vi "Shutdown DUT.vi"(7 "0x01 (F)":bool, 8 "error in (no error)":errorcluster, 9 "Device On?":bool, 10 "Blast?":bool, 11 "Data In":T1={"Message"="", "Homed?"=FALSE, "NextState"=enum."Timeout", "G.Load"=0.0, "G.Position"=0.0, "Load#"=0, "[G.Loads]"=[], "[TotalLoads]"=[], "[Errors]"=[], "ZeroWait"=0, "Results"=[], "DwellWait"=FALSE, "Test Result"=FALSE, "[CondyleLoads]"=[], "[Max]"=[], "[Min]"=[], "Valid String?"=FALSE, "ScanTime"=timestamp(0 s since 1904-01-01), "ScannedString"="", "LabelDevID"=0, "MfgDate"=timestamp(0 s since 1904-01-01), "[EEPROM Cmds]"=[], "[CalData]"=[], "[A/Ds]"=[], "[A/Dmax]"=[], "[A/Dmin]"=[], "BattMax"=0.0, "BattMin"=0.0, "DwellTime"=2000, "PendingDeviceType"="", "Zero G.load"=0.0, "GAINC Value"="", "Programming Step"=enum."Load EEPROM", "Front Panel Program?"=FALSE, "Final Program?"=FALSE, "PCB Score"=100, "AssyScore"=100, "Pass/Fail #"="", "Result String"="", "Programming Mode"=enum."Initial Program", "Angle Test Step"=enum."Initialize", "Accel Values"=[], "Shutdown Counter"=0, "V1"=0, "V2"=0, "V3"=0, "V4"=0, "EEPROM Data"=[], "Counter"=0, "Page#"=0, "Timer"=timestamp(0 s since 1904-01-01), "Use Mark10?"=FALSE, "Eng-Result#"=0, "DUT Serial #"=0, "Scroll Message?"=FALSE, "Clear Message"=FALSE, "Batt Test Step "=enum."Initialize", "RXTX Window Found?"=FALSE, "Shutdown First Call?"=FALSE, "A2 Delay (msec)"=500, "Support Script"={"Script #"="", "Script Revision"="", "[OEMs]"=[], "[[DeviceTypes]]"=[], "[[DeviceTypesVals]]"=[], "[[List of Errors]]"=[], "Default GAINC"="", "[[ASICtrims]]"=[], "ID For Echo"="", "Condyle A CalFactor"=100, "Condyle B CalFactor"=100, "[OEMs Prefix]"=[], "Packet ID 18"="", "[[Force Table Load Test]]"=[], "[[Force Table AccurTest]]"=[]}, "Serial Table"={"Serial File Path"=path "", "[[Serial Lookup Table]]"=[], "Serial Device Info"=[], "Valid Serial?"=FALSE}, "Target Information"={"Target Brand"="", "Target DeviceType"="", "Target Serial#"=100, "Target Lot#"=0, "Target DevID"=0, "Target Channel"=5}, "Operator"="", "COM Port"="", "Config Path"=path "", "Tx Array"=[], "DUT Parameters"={"Channel"=0, "DeviceID"=0, "Script Rev"=0, "Month"=0, "Day"=0, "Year"=0, "Lot#"=0, "V1"=0, "V2"=0, "V3"=0, "V4"=0, "MFG"=0, "Cal FactorA 10"=0, "Cal FactorB 10  "=0, "Cal FactorA 16"=0, "Cal FactorB 16"=0, "ASICtrim"=[], "TmpChan"=0, "GAINC"="", "Brand"="", "Device"="", "Serial #"=0, "Batt310"=0, "Batt 280"=0}, "FTS Main?"=FALSE, "Loading"={"[Forces]"=[], "[Dwell]"=[], "Loading Step"=enum."Initialize Test"}, "Software Version"="", "Correction Factor"="", "Second Load Test"=FALSE, "Acc Loads"=[], "Mark10 Config"={"H2S%"=[80.0, 85.0, 90.0, 95.0, 100.0], "H2S Speed"=[12.0, 8.0, 6.0, 4.0, 2.0], "H to S"=2.0, "Home Speed"=1.0, "LoadWin"=0.0, "Load Speed"=0.0, "PID"={"Kp"=0.04, "Kd"=0.005001, "Ki"=2.9999999999999923e-05}}, "Channels"={"Transceiver Ch"=5, "Operating Ch"=5, "Start Ch"=0}, "Channel EEPROM"=[], "Load Notes"=[], "Engr Log?"=FALSE, "Time"=[], "Program Retry"=FALSE, "Operator Channel"="", "Target Channel "="", "New Data Program"=FALSE, "NFHU Pass?"=FALSE, "Cycle Number"=0, "Cal Cycle#"=0, "[Avg G.Loads] "=[], "[Avg A/Ds] "=[], "Cal Retry?"=FALSE, "[Total A/Ds]  "=[], "Cycle Num LA"=0, "LA Cycle# "=0, "Shim Num"=0, "Shim#  "=0, "Angle Test?"=FALSE} {"Mark10 Config"."PID"."Ki" min=0.0 max=200.0 format="%.6f"; "Mark10 Config"."PID"."Kd" min=0.0 max=200.0 format="%.6f"; "Mark10 Config"."PID"."Kp" min=0.0 max=200.0 format="%.6f"; "DUT Parameters"."ASICtrim" format="%02x"}) -> (0 "error out":errorcluster, 3 "State-machine Local Variables out":T1={"Message"="", "Homed?"=FALSE, "NextState"=enum."Timeout", "G.Load"=0.0, "G.Position"=0.0, "Load#"=0, "[G.Loads]"=[], "[TotalLoads]"=[], "[Errors]"=[], "ZeroWait"=0, "Results"=[], "DwellWait"=FALSE, "Test Result"=FALSE, "[CondyleLoads]"=[], "[Max]"=[], "[Min]"=[], "Valid String?"=FALSE, "ScanTime"=timestamp(0 s since 1904-01-01), "ScannedString"="", "LabelDevID"=0, "MfgDate"=timestamp(0 s since 1904-01-01), "[EEPROM Cmds]"=[], "[CalData]"=[], "[A/Ds]"=[], "[A/Dmax]"=[], "[A/Dmin]"=[], "BattMax"=0.0, "BattMin"=0.0, "DwellTime"=2000, "PendingDeviceType"="", "Zero G.load"=0.0, "GAINC Value"="", "Programming Step"=enum."Load EEPROM", "Front Panel Program?"=FALSE, "Final Program?"=FALSE, "PCB Score"=100, "AssyScore"=100, "Pass/Fail #"="", "Result String"="", "Programming Mode"=enum."Initial Program", "Angle Test Step"=enum."Initialize", "Accel Values"=[], "Shutdown Counter"=0, "V1"=0, "V2"=0, "V3"=0, "V4"=0, "EEPROM Data"=[], "Counter"=0, "Page#"=0, "Timer"=timestamp(0 s since 1904-01-01), "Use Mark10?"=FALSE, "Eng-Result#"=0, "DUT Serial #"=0, "Scroll Message?"=FALSE, "Clear Message"=FALSE, "Batt Test Step "=enum."Initialize", "RXTX Window Found?"=FALSE, "Shutdown First Call?"=FALSE, "A2 Delay (msec)"=500, "Support Script"={"Script #"="", "Script Revision"="", "[OEMs]"=[], "[[DeviceTypes]]"=[], "[[DeviceTypesVals]]"=[], "[[List of Errors]]"=[], "Default GAINC"="", "[[ASICtrims]]"=[], "ID For Echo"="", "Condyle A CalFactor"=100, "Condyle B CalFactor"=100, "[OEMs Prefix]"=[], "Packet ID 18"="", "[[Force Table Load Test]]"=[], "[[Force Table AccurTest]]"=[]}, "Serial Table"={"Serial File Path"=path "", "[[Serial Lookup Table]]"=[], "Serial Device Info"=[], "Valid Serial?"=FALSE}, "Target Information"={"Target Brand"="", "Target DeviceType"="", "Target Serial#"=100, "Target Lot#"=0, "Target DevID"=0, "Target Channel"=5}, "Operator"="", "COM Port"="", "Config Path"=path "", "Tx Array"=[], "DUT Parameters"={"Channel"=0, "DeviceID"=0, "Script Rev"=0, "Month"=0, "Day"=0, "Year"=0, "Lot#"=0, "V1"=0, "V2"=0, "V3"=0, "V4"=0, "MFG"=0, "Cal FactorA 10"=0, "Cal FactorB 10  "=0, "Cal FactorA 16"=0, "Cal FactorB 16"=0, "ASICtrim"=[], "TmpChan"=0, "GAINC"="", "Brand"="", "Device"="", "Serial #"=0, "Batt310"=0, "Batt 280"=0}, "FTS Main?"=FALSE, "Loading"={"[Forces]"=[], "[Dwell]"=[], "Loading Step"=enum."Initialize Test"}, "Software Version"="", "Correction Factor"="", "Second Load Test"=FALSE, "Acc Loads"=[], "Mark10 Config"={"H2S%"=[80.0, 85.0, 90.0, 95.0, 100.0], "H2S Speed"=[12.0, 8.0, 6.0, 4.0, 2.0], "H to S"=2.0, "Home Speed"=1.0, "LoadWin"=0.0, "Load Speed"=0.0, "PID"={"Kp"=0.04, "Kd"=0.005001, "Ki"=2.9999999999999923e-05}}, "Channels"={"Transceiver Ch"=5, "Operating Ch"=5, "Start Ch"=0}, "Channel EEPROM"=[], "Load Notes"=[], "Engr Log?"=FALSE, "Time"=[], "Program Retry"=FALSE, "Operator Channel"="", "Target Channel "="", "New Data Program"=FALSE, "NFHU Pass?"=FALSE, "Cycle Number"=0, "Cal Cycle#"=0, "[Avg G.Loads] "=[], "[Avg A/Ds] "=[], "Cal Retry?"=FALSE, "[Total A/Ds]  "=[], "Cycle Num LA"=0, "LA Cycle# "=0, "Shim Num"=0, "Shim#  "=0, "Angle Test?"=FALSE} {"Mark10 Config"."PID"."Ki" min=0.0 max=200.0 format="%.6f"; "Mark10 Config"."PID"."Kd" min=0.0 max=200.0 format="%.6f"; "Mark10 Config"."PID"."Kp" min=0.0 max=200.0 format="%.6f"; "DUT Parameters"."ASICtrim" format="%02x"})   [LabVIEW 2015]
uses:
  Controls/LocalVars.ctl
  Controls/Gen2 FT states.ctl
  Controls/Iniial Device Programming.ctl
  ProgramStageControl.ctl
  Controls/Batt Cap Steps.ctl
  Controls/Support Script.ctl
  Controls/Serial Table.ctl
  Controls/Device Information.ctl
  Controls/InfoPacket.ctl
  Controls/Loading.ctl
  Controls/Load Step.ctl
  Controls/Mark10 Config.ctl
  Controls/PID parameters.ctl
  Controls/Channels.ctl
  RxTx/XceiverCmds.ctl
  Controls/Gen2 FT Globals.vi
panel:
  out "Numeric":i32
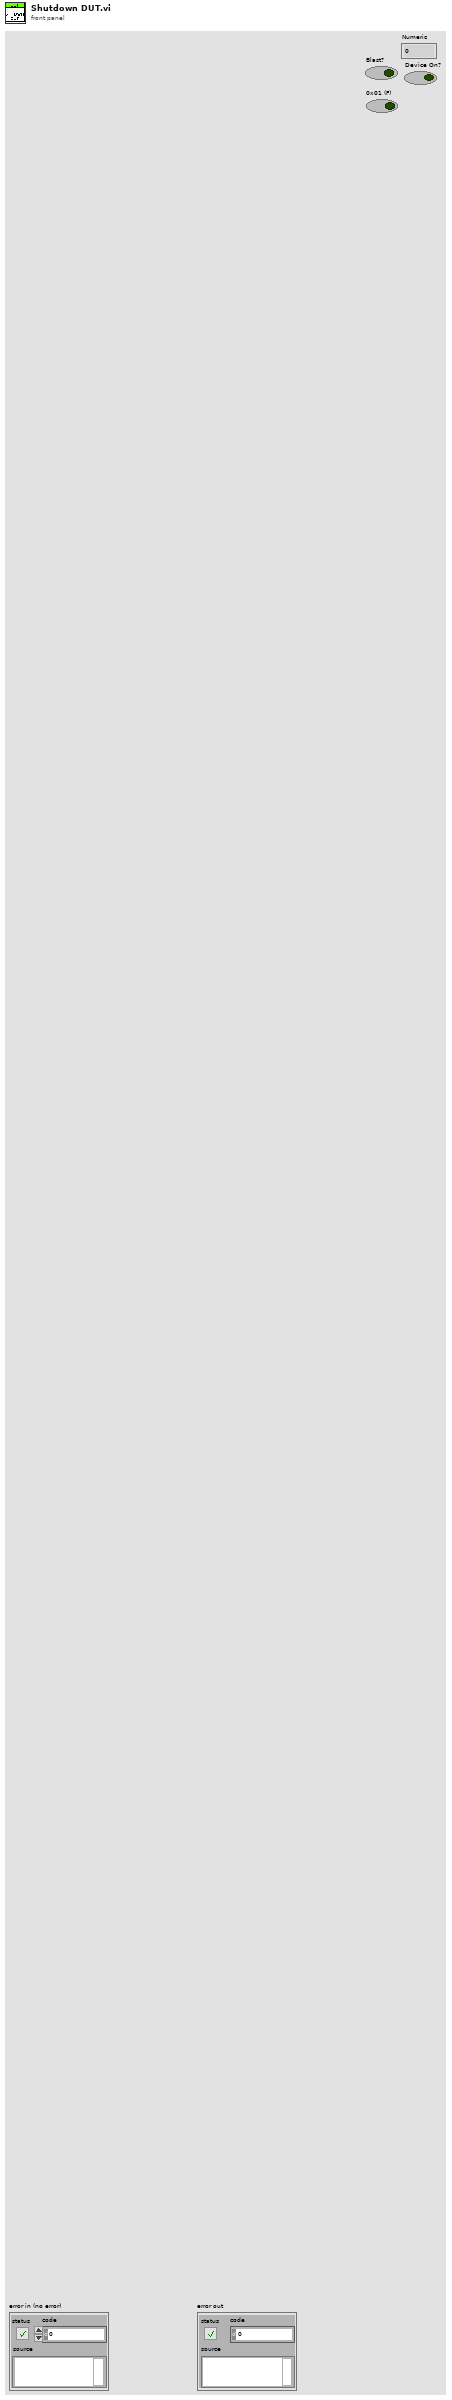
[diagram p1: front panel]
types:
  T1 = typedef "LocalVars.ctl" = cluster{"Message":string, "Homed?":bool, "NextState":T2, "G.Load":dbl, "G.Position":dbl, "Load#":i32, "[G.Loads]":dbl[], "[TotalLoads]":dbl[], "[Errors]":dbl[][], "ZeroWait":u32, "Results":dbl[], "DwellWait":bool, "Test Result":bool, "[CondyleLoads]":dbl[][], "[Max]":dbl[], "[Min]":dbl[], "Valid String?":bool, "ScanTime":timestamp, "ScannedString":string, "LabelDevID":u32, "MfgDate":timestamp, "[EEPROM Cmds]":u8[][], "[CalData]":u8[][], "[A/Ds]":dbl[][], "[A/Dmax]":dbl[], "[A/Dmin]":dbl[], "BattMax":dbl, "BattMin":dbl, "DwellTime":i32, "PendingDeviceType":string, "Zero G.load":dbl, "GAINC Value":string, "Programming Step":T3, "Front Panel Program?":bool, "Final Program?":bool, "PCB Score":i32, "AssyScore":i32, "Pass/Fail #":string, "Result String":string, "Programming Mode":T4, "Angle Test Step":enum16{"Initialize", "Get X", "Get Y", "Get Z", "Next Test"}, "Accel Values":dbl[][], "Shutdown Counter":u32, "V1":i32, "V2":i32, "V3":i32, "V4":i32, "EEPROM Data":i32[][], "Counter":i32, "Page#":i32, "Timer":timestamp, "Use Mark10?":bool, "Eng-Result#":u32, "DUT Serial #":i32, "Scroll Message?":bool, "Clear Message":bool, "Batt Test Step ":T5, "RXTX Window Found?":bool, "Shutdown First Call?":bool, "A2 Delay (msec)":i16, "Support Script":T6, "Serial Table":T7, "Target Information":T8, "Operator":string, "COM Port":string, "Config Path":path, "Tx Array":u8[], "DUT Parameters":T9, "FTS Main?":bool, "Loading":T10, "Software Version":string, "Correction Factor":string, "Second Load Test":bool, "Acc Loads":dbl[][], "Mark10 Config":T12, "Channels":T14, "Channel EEPROM":i32[][], "Load Notes":string[], "Engr Log?":bool, "Time":timestamp[], "Program Retry":bool, "Operator Channel":string, "Target Channel ":string, "New Data Program":bool, "NFHU Pass?":bool, "Cycle Number":i32, "Cal Cycle#":i32, "[Avg G.Loads] ":dbl[], "[Avg A/Ds] ":dbl[][], "Cal Retry?":bool, "[Total A/Ds]  ":dbl[][], "Cycle Num LA":i32, "LA Cycle# ":i32, "Shim Num":i32, "Shim#  ":i32, "Angle Test?":bool}
  T2 = typedef "Gen2 FT states.ctl" = enum16{"---------SETUP-------", "Initialization", "Read Support Data", "Initialize Mark-10", "Initialize Transceiver", "------UTILITIES------", "Change DUT Channel", "Find RxTx Window", "Reset Device", "Scan Channels", "Read Serial Lookup", "Shutdown Device", "ESTOP", "--------USER---------", "Timeout", "-----PROGRAM-----", "Program Device", "------MARK10--------", "Go Home", "MoveUp", "MoveDown", "Goto Load", "Goto Position", "Stop Motor", "---------TESTS--------", "Start Test", "Angle Test", "Load Test", "Load Accuracy Test", "Battery Test", "------RESULTS-------", "End Test", "Display Result", "--------EXIT--------", "Exit"}
  T3 = typedef "Iniial Device Programming.ctl" = enum16{"Load EEPROM", "Send First A1", "Send EEPROM", "Send A1", "Check EEPROM Echo", "Verify transmission", "Programming Successful", "Programming Failed"}
  T4 = typedef "ProgramStageControl.ctl" = enum16{"Initial Program", "GainC", "Scales"}
  T5 = typedef "Batt Cap Steps.ctl" = enum16{"Initialize", "Collect 2.8 Volts", "Collect 3.1 Volts", "Check Results"}
  T6 = typedef "Support Script.ctl" = cluster{"Script #":string, "Script Revision":string, "[OEMs]":string[], "[[DeviceTypes]]":string[][], "[[DeviceTypesVals]]":u16[][], "[[List of Errors]]":string[][], "Default GAINC":string, "[[ASICtrims]]":u8[][], "ID For Echo":string, "Condyle A CalFactor":i32, "Condyle B CalFactor":i32, "[OEMs Prefix]":string[], "Packet ID 18":string, "[[Force Table Load Test]]":dbl[][], "[[Force Table AccurTest]]":dbl[][]}
  T7 = typedef "Serial Table.ctl" = cluster{"Serial File Path":path, "[[Serial Lookup Table]]":string[][], "Serial Device Info":string[], "Valid Serial?":bool}
  T8 = typedef "Device Information.ctl" = cluster{"Target Brand":string, "Target DeviceType":string, "Target Serial#":i32, "Target Lot#":u32, "Target DevID":u32, "Target Channel":u8}
  T9 = typedef "InfoPacket.ctl" = cluster{"Channel":u8, "DeviceID":u32, "Script Rev":u8, "Month":u8, "Day":u8, "Year":u8, "Lot#":u32, "V1":u16, "V2":u16, "V3":u16, "V4":u16, "MFG":u8, "Cal FactorA 10":u8, "Cal FactorB 10  ":u8, "Cal FactorA 16":u8, "Cal FactorB 16":u8, "ASICtrim":u8[], "TmpChan":u8, "GAINC":string, "Brand":string, "Device":string, "Serial #":u64, "Batt310":u16, "Batt 280":u16}
  T10 = typedef "Loading.ctl" = cluster{"[Forces]":dbl[], "[Dwell]":dbl[], "Loading Step":T11}
  T11 = typedef "Load Step.ctl" = enum16{"Initialize Test", "Go Home", "Detect Dev Surface", "Wait to zero Device", "Zero Device", "Do Test", "Test Result"}
  T12 = typedef "Mark10 Config.ctl" = cluster{"H2S%":dbl[], "H2S Speed":dbl[], "H to S":dbl, "Home Speed":dbl, "LoadWin":dbl, "Load Speed":dbl, "PID":T13}
  T13 = typedef "PID parameters.ctl" = cluster{"Kp":dbl, "Kd":dbl, "Ki":dbl}
  T14 = typedef "Channels.ctl" = cluster{"Transceiver Ch":u8, "Operating Ch":u8, "Start Ch":u8}
  T15 = typedef "XceiverCmds.ctl" = enum8{"Get Window", "Set Window", "Load&Xmit", "Find Window", "Load CC1101", "Blink LED1", "Blink LED2", "Gen2 Mode", "Request Rev", "Gen2 Mode & Req Rev", "Load Device Settings", "Reset Xceiver", "Set Channel", "Read Channel"}
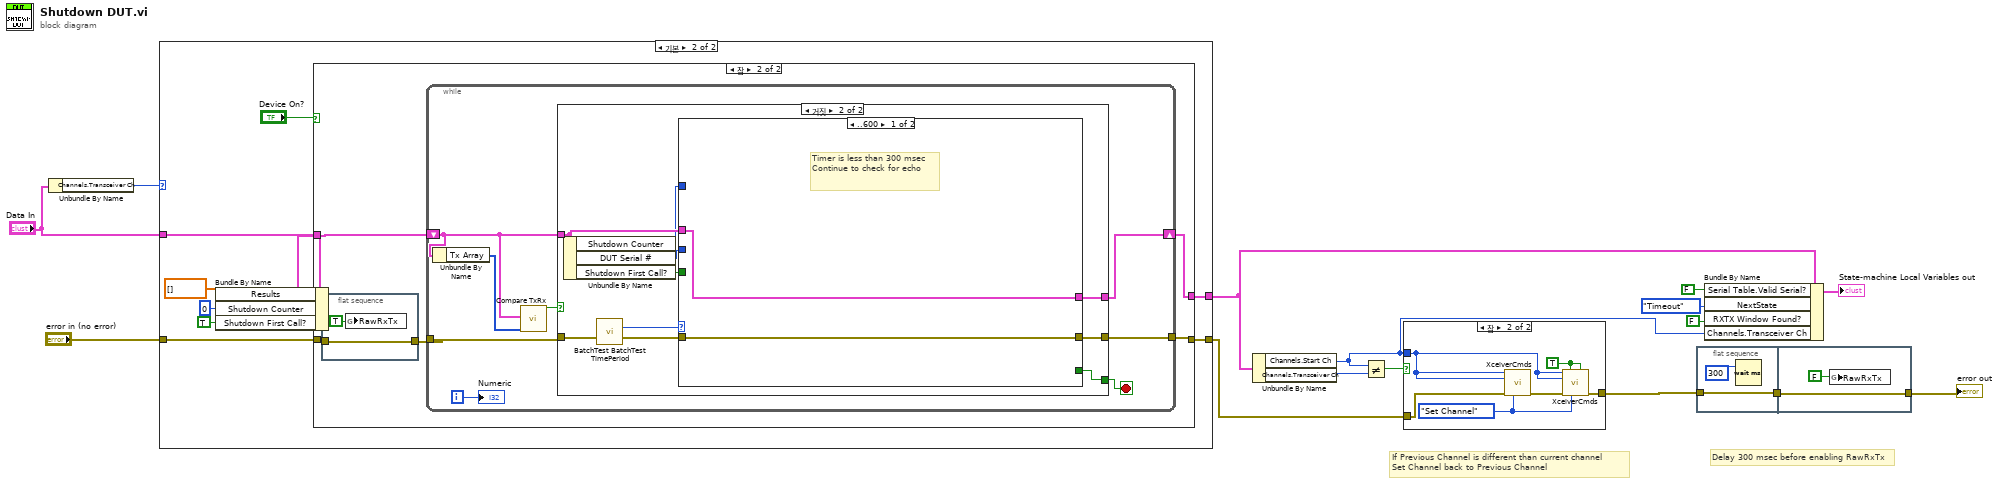
[diagram p0: block diagram]
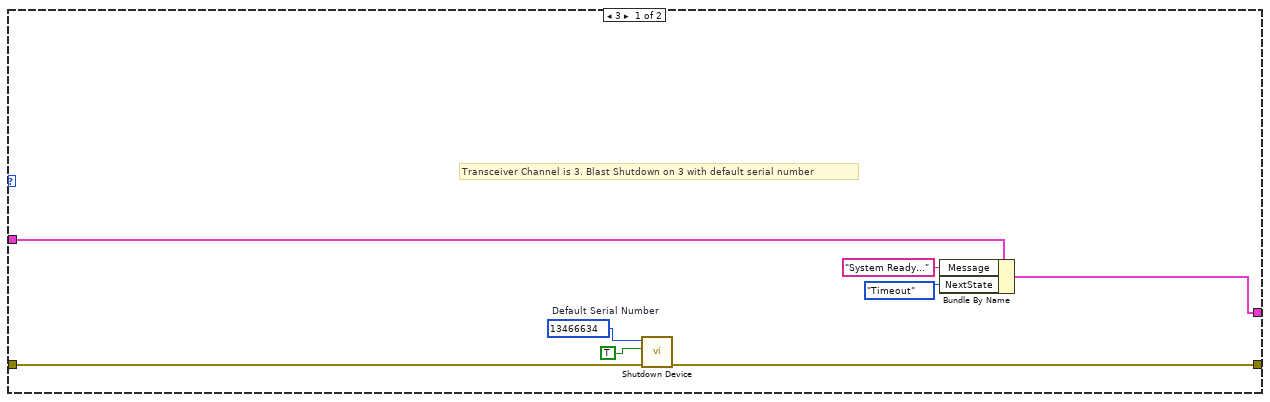
[diagram p3: hidden frame]
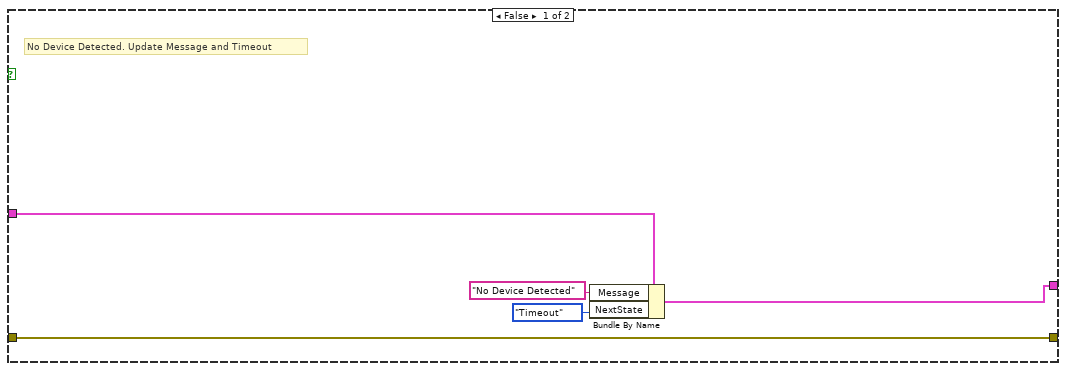
[diagram p4: hidden frame]
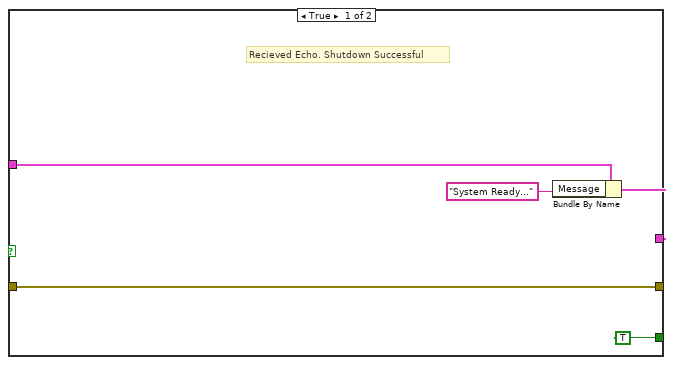
[diagram p5: hidden frame]
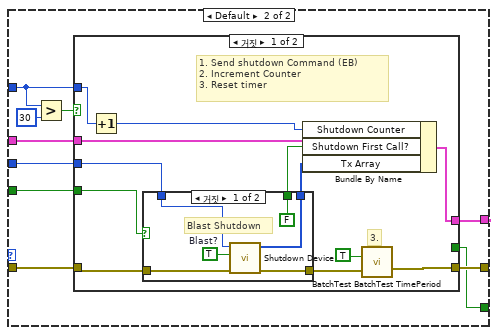
[diagram p6: hidden frame]
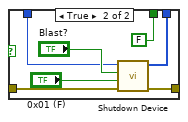
[diagram p7: hidden frame]
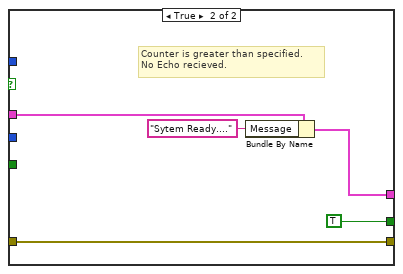
[diagram p8: hidden frame]
diagram:
  # "Delay 300 msec before enabling RawRxTx"
  # "If Previous Channel is different than current channel\nSet Channel back to Previous Channel"
  n1 = Unbundle By Name("Data In") -> ("Channels.Transceiver Ch"=w13:u8)
  n2 = case shown="기본" w13 {
    tunnel: "error in (no error)" -> [w21 w29]
    tunnel: [w20 w32] -> w6
    tunnel: "Data In" -> [w23 w31]
    tunnel: [w19 w30] -> w10
    frame 3 {
      w22 = u32 13466634  # Default Serial Number
      # "Transceiver Channel is 3. Blast Shutdown on 3 with default serial number"
      n3 = call "Shutdown Device.vi"("error in (no error)"=w21, "Blast? (F)"=TRUE ("Blast?"), "Serial Number"=w22) -> ("error out"=w20:errorcluster)  [unwired: 7 in, 1 out]
      n4 = Bundle By Name(cluster=w23, "Message"="System Ready...", "NextState"=Gen2_FT_states."Timeout") -> (w19:T1)
    }
    frame Default {
      n5 = Bundle By Name(cluster=w31, "Results"=dbl[] [], "Shutdown Counter"=u32 0, "Shutdown First Call?"=TRUE) -> (w26:T1)
      n6 = case shown="참" "Device On?" {
        tunnel: w29 -> [w37 w42]
        tunnel: [w37 w38] -> w32
        tunnel: [w35 w39] -> w30
        tunnel: w26 -> [w36 w40]
        frame False {
          # "No Device Detected. Update Message and Timeout"
          n7 = Bundle By Name(cluster=w36, "Message"="No Device Detected", "NextState"=Gen2_FT_states."Timeout") -> (w35:T1)
        }
        frame True {
          n8 = flat-sequence {
            tunnel: w42 -> [w43]
            tunnel: [w43] -> w41
            frame #0 {
              n9 = global write "Gen2 FT Globals.vi" "RawRxTx"(TRUE ("RawRxTx")) -> ()
            }
          }
          n10 = while {
            tunnel: w41 -> [w45]
            tunnel: [w51] -> w38
            shift-right: [w52] -> w39
            shift-left: w40 -> [w48]
            i -> [w49]
            stop <- w50 stop-if-true
            n11 = Unbundle By Name(w48) -> ("Tx Array"=w47:u8[])
            n12 = call "Compare TxRx.vi"("RawTx"=w47, "Data Cluster In"=w48) -> ("0x80 + Content?"=w46:bool)  [unwired: 7 in, 2 out]
            n13 = case shown="거짓" w46 {
              tunnel: [w57 w66] -> w52
              tunnel: w48 -> [w54 w64]
              tunnel: [w53 w62] -> w51
              tunnel: w45 -> [w53 w67]
              tunnel: [TRUE ("Done?") w60] -> w50
              frame True {
                # "Recieved Echo. Shutdown Successful"
                n14 = Bundle By Name(cluster=w54, "Message"="System Ready...") -> (w57:T1)
              }
              frame False {
                n15 = Unbundle By Name(w64) -> ("Shutdown Counter"=w59:u32, "DUT Serial #"=w61:i32, "Shutdown First Call?"=w58:bool)
                n16 = call "BatchTest BatchTest TimePeriod.vi"("error in (no error)"=w67) -> ("Time(mS)"=w65:u32, "error out"=w63:errorcluster)  [unwired: 13 in]
                n17 = case shown="..600" w65 {
                  tunnel: w64 -> [w68 w77]
                  tunnel: [w68 w76] -> w66
                  tunnel: w63 -> [w69 w75]
                  tunnel: [w69 w74] -> w62
                  tunnel: w61 -> [_ w73]
                  tunnel: [_ w72] -> w60
                  tunnel: w59 -> [_ w71]
                  tunnel: w58 -> [_ w70]
                  frame ..600 {
                    # "Timer is less than 300 msec\nContinue to check for echo"
                  }
                  frame Default {
                    n18 = Greater?(x=w71, y=u32 30) -> (0:w78:bool)
                    n19 = case shown="거짓" w78 {
                      tunnel: w77 -> [w90 w109]
                      tunnel: [w88 w108] -> w76
                      tunnel: w75 -> [w85 w105]
                      tunnel: [w89 w105] -> w74
                      tunnel: w71 -> [w87 _]
                      tunnel: w73 -> [w83 _]
                      tunnel: [_ TRUE] -> w72
                      tunnel: w70 -> [w82 _]
                      frame False {
                        # "3."
                        # "1. Send shutdown Command (EB) \n2. Increment Counter\n3. Reset timer"
                        n20 = Increment(x=w87) -> (x+1=w86:u32)
                        n21 = case shown="거짓" w82 {
                          tunnel: w85 -> [w95 w104]
                          tunnel: [w94 w103] -> w84
                          tunnel: w83 -> [w93 w101]
                          tunnel: [FALSE ("Shutdown First Call?") FALSE ("Shutdown First Call?")] -> w81
                          tunnel: [w92 w98] -> w80
                          frame False {
                            w96 = TRUE  # Blast?
                            # "Blast Shutdown"
                            n22 = call "Shutdown Device.vi"("error in (no error)"=w95, "Blast? (F)"=w96, "Serial Number"=w93) -> ("error out"=w94:errorcluster, "Tx array"=w92:u8[])  [unwired: 7 in]
                          }
                          frame True {
                            n23 = call "Shutdown Device.vi"("error in (no error)"=w104, "01 Command? (F)"="0x01 (F)", "Blast? (F)"="Blast?", "Serial Number"=w101) -> ("error out"=w103:errorcluster, "Tx array"=w98:u8[])  [unwired: 6 in]
                          }
                        }
                        n24 = Bundle By Name(cluster=w90, "Shutdown Counter"=w86, "Shutdown First Call?"=w81, "Tx Array"=w80) -> (w88:T1)
                        n25 = call "BatchTest BatchTest TimePeriod.vi"("Initialize?"=TRUE, "error in (no error)"=w84) -> ("error out"=w89:errorcluster)  [unwired: 12 in, 1 out]
                      }
                      frame True {
                        # "Counter is greater than specified. \nNo Echo recieved."
                        n26 = Bundle By Name(cluster=w109, "Message"="Sytem Ready....") -> (w108:T1)
                      }
                    }
                  }
                }
              }
            }
            "Numeric" <- w49
          }
        }
      }
    }
  }
  n27 = Unbundle By Name(w10) -> ("Channels.Start Ch"=w1:u8, "Channels.Transceiver Ch"=w11:u8)
  n28 = Not Equal?(x=w1, y=w11) -> (x != y?=w12:bool)
  n29 = case shown="참" w12 {
    tunnel: w1 -> [_ w112]
    tunnel: [w110 w113] -> w4
    tunnel: w6 -> [w110 w111]
    frame False {
    }
    frame True {
      w116 = TRUE ("RF Chip0 Enable")
      w115 = XceiverCmds."Set Channel" ("XceiverCmd")
      n30 = call "XceiverCmds.vi"("RF Chip0 Channel"=w112, "RF Chip1 Channel"=w112, "error in (no error)"=w111, "XceiverCmd"=w115) -> ("error out"=w114:errorcluster)  [unwired: 9 in, 2 out]
      n31 = call "XceiverCmds.vi"("RF Chip0 Channel"=w112, "RF Chip0 Enable"=w116, "RF Chip1 Enable"=w116, "RF Chip1 Channel"=w112, "error in (no error)"=w114, "XceiverCmd"=w115) -> ("error out"=w113:errorcluster)  [unwired: 7 in, 2 out]
    }
  }
  n32 = flat-sequence {
    tunnel: [w117] -> w5
    tunnel: w4 -> [w117]
    tunnel: w5 -> [w120]
    tunnel: [w120] -> w3
    frame #0 {
      n33 = Wait (ms)(milliseconds to wait=u32 300) -> ()  [unwired: 1 out]
    }
    frame #1 {
      n34 = global write "Gen2 FT Globals.vi" "RawRxTx"(FALSE ("RawRxTx")) -> ()
    }
  }
  n35 = Bundle By Name(cluster=w10, "Serial Table.Valid Serial?"=FALSE, "NextState"=Gen2_FT_states."Timeout", "RXTX Window Found?"=FALSE, "Channels.Transceiver Ch"=w1) -> (→"State-machine Local Variables out":T1)
  "error out" <- w3
